vi "GetLogFromErrorManager.vi"(8 "error in (no error)":errorcluster, 11 "CDependencyInspection in":refnum<class "CDependencyInspection.lvclass">) -> (0 "error out":errorcluster, 1 "Log results":string[][](array[string]), 3 "CDependencyInspection out":refnum<class "CDependencyInspection.lvclass">)   [LabVIEW 2020, in "DependencyInspection.lvlib" / "CDependencyInspection.lvclass"]
uses:
  CDependencyInspection.lvclass
  CDependencyInspection.lvclass/CDependencyInspection.ctl
  obj/Addons/ErrorManager.lvlibp/ErrorManager/ErrorManager.lvclass
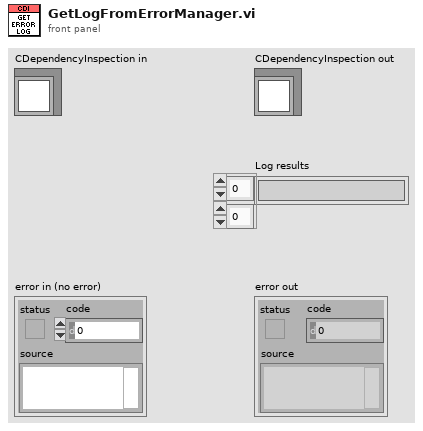
[diagram p1: front panel]
types:
  T1 = typedef "ErrorManager.lvlibp/ErrorManager.lvclass/ErrorInfo.ctl" = cluster{"Time Stamp":timestamp, "Message":string, "Type":T2}
  T2 = typedef "LabVIEWObjectInterfaces.lvlibp/IErrorManager.lvclass/ErrorType.ctl" = enum16{"Info", "Warning", "Error"}
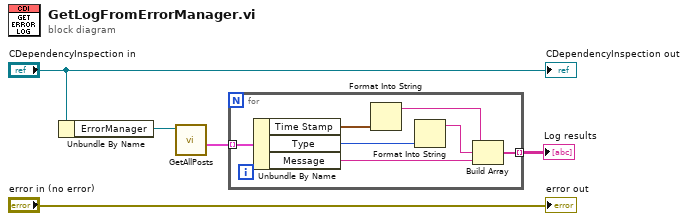
[diagram p0: block diagram]
diagram:
  n1 = Unbundle By Name("CDependencyInspection in") -> ("ErrorManager"=w3:refnum<class "ErrorManager.lvclass">)
  n2 = call-dynamic "GetAllPosts.vi"("ErrorManager in"=w3) -> ("Errors"=w2:T1[])  [unwired: 8 in, 2 out]
  n3 = for {
    tunnel: w2 -> [w12] mode=indexing
    tunnel: [w6] -> w1 mode=indexing
    n4 = Unbundle By Name(w12) -> ("Time Stamp"=w11:timestamp, "Type"=w10:T2, "Message"=w8:string)
    n5 = Format Into String(w11) -> (resulting string=w9:string)  [unwired: 3 in, 1 out]
    n6 = Format Into String(w10) -> (resulting string=w7:string)  [unwired: 3 in, 1 out]
    n7 = Build Array(w9, w7, w8) -> (w6:string[])
  }
  "Log results" <- w1
  "error out" <- "error in (no error)"
  "CDependencyInspection out" <- "CDependencyInspection in"
